vi "current monitor4.vi"() -> ()   [LabVIEW 2010]
uses:
  <vilib>/Utility/file.llb/Write To Spreadsheet File (DBL).vi
  <userlib>/Nanonis Prog Interface V5/Nanonis Prog Interface.lvlib
panel:
  out "Averaged":cluster{"f0":dbl, "df":dbl, dbl[]}(graph)
  out "Start Time":string
  in  "Number of Loops":dbl
  in  "Start":bool
  in  "Loop delay":dbl
  out "error out":errorcluster
  in  "Path":path
  out "Spectrum Analyzer":cluster{"f0":dbl, "df":dbl, "values":dbl[]}(graph)
  out "Current (A)":sgl format="%#_6p"
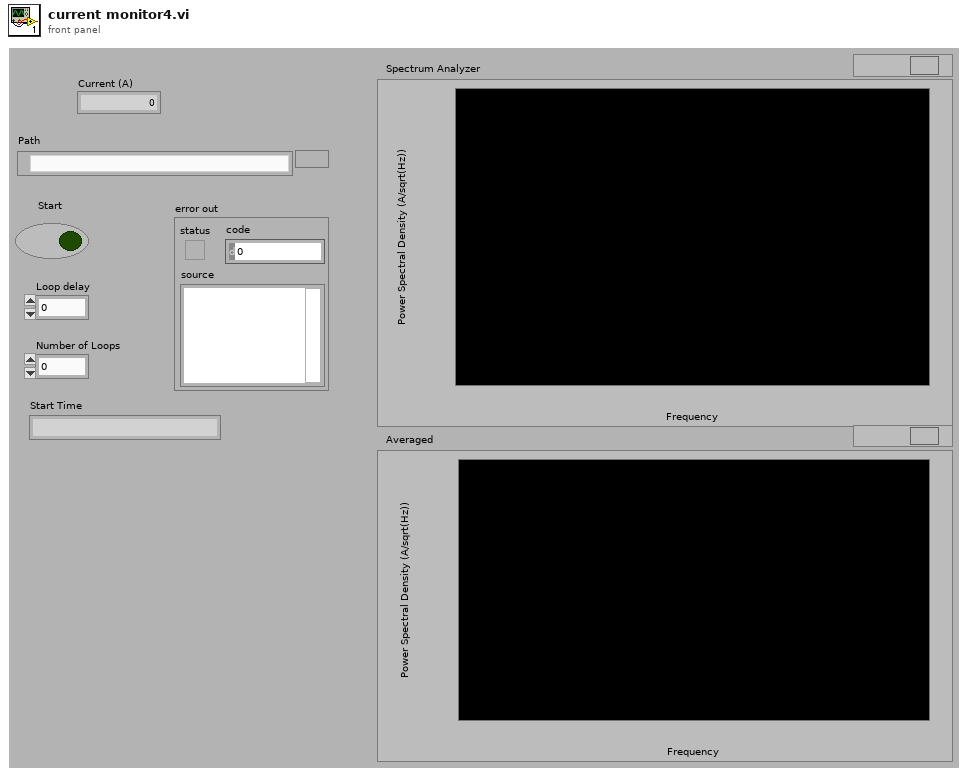
[diagram p1: front panel]
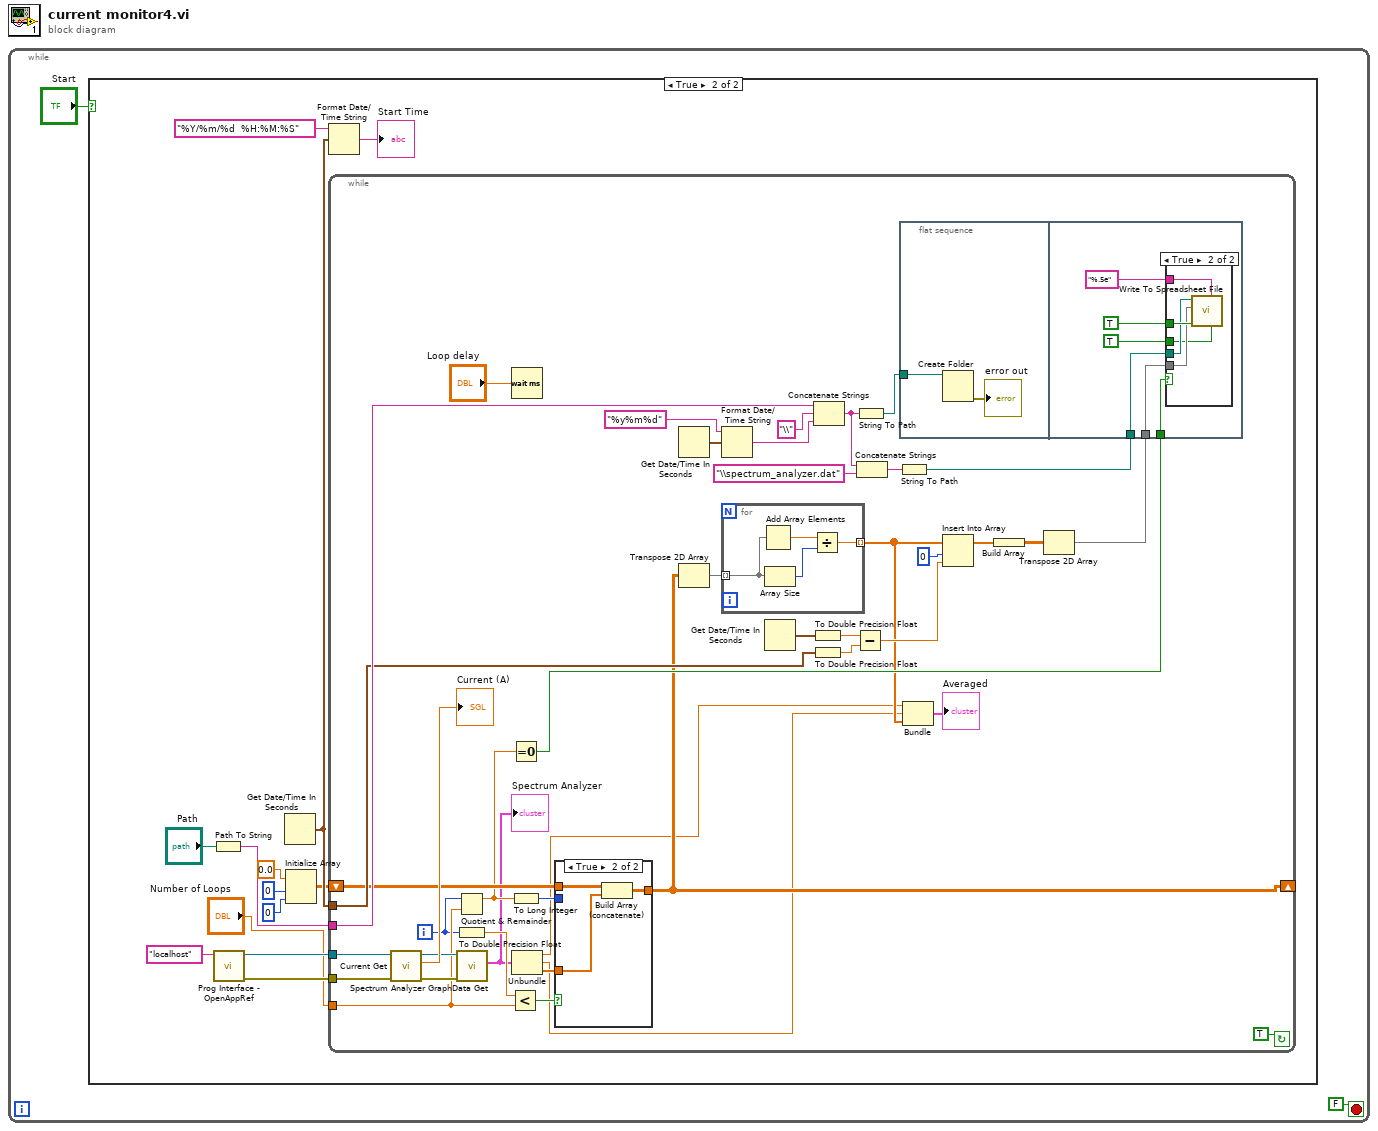
[diagram p0: block diagram]
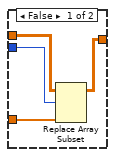
[diagram p3: hidden frame]
diagram:
  n1 = while {
    stop <- FALSE stop-if-true
    n2 = case shown="True" "Start" {
      frame False {
      }
      frame True {
        n3 = Path To String(path="Path") -> (string=w11:string)
        n4 = call <userlib>:"Prog Interface - OpenAppRef.vi"("Machine name (local machine IP)"="localhost" ("machine name (localhost)")) -> ("Error out"=w14:errorcluster, "Application reference"=w15:refnum<vi>)  [unwired: 5 in]
        n5 = Get Date/Time In Seconds() -> (seconds since 1Jan1904=w9:timestamp)
        n6 = Initialize Array(0.0, 0, 0) -> (w3:dbl[][])
        n7 = Format Date/Time String(time format string (%c)="%Y/%m/%d  %H:%M:%S", seconds (now)=w9) -> (date/time string=→"Start Time":string)  [unwired: 1 in]
        n8 = while {
          tunnel: w15 -> [w57]
          tunnel: w14 -> [w56]
          tunnel: w11 -> [w49]
          tunnel: w9 -> [w35]
          tunnel: "Number of Loops" -> [w30]
          shift-right: [w24] -> _
          shift-left: w3 -> [w27]
          i -> [w26]
          stop <- TRUE continue-if-true
          n9 = call <userlib>:"Current Get.vi"("Error in (no error)"=w56, "Application ref in"=w57) -> ("Error out"=w53:errorcluster, "Current (A)"=→"Current (A)":sgl, "Application ref out"=w54:refnum<vi>)  [unwired: 5 in]
          n10 = Quotient & Remainder(x=w26, y=w30) -> (x-y*floor(x/y)=w21:dbl)  [unwired: 1 out]
          n11 = To Double Precision Float(number=w26) -> (double precision float=w29:dbl)
          n12 = call <userlib>:"Spectrum Analyzer GraphData Get.vi"("Error in (no error)"=w53, "Application ref in"=w54) -> ("FFT data"=w20:cluster{"f0":dbl, "df":dbl, "values":dbl[]})  [unwired: 7 in, 2 out]
          "Spectrum Analyzer" <- w20
          n13 = Less?(x=w29, y=w30) -> (x < y?=w31:bool)
          n14 = Equal To 0?(x=w21) -> (x = 0?=w41:bool)
          n15 = To Long Integer(number=w21) -> (32bit integer=w22:i32)
          n16 = Wait (ms)(milliseconds to wait="Loop delay") -> ()  [unwired: 1 out]
          n17 = Unbundle(w20) -> ("f0"=w17:dbl, "df"=w16:dbl, "values"=w28:dbl[])
          n18 = case shown="True" w31 {
            tunnel: w28 -> [w63 w68]
            tunnel: [w64 w67] -> w24
            tunnel: w27 -> [w65 w66]
            tunnel: w22 -> [w62 _]
            frame False {
              n19 = Replace Array Subset(array=w65, new element=w63, index (row)=w62) -> (w64:dbl[][])  [unwired: 1 in]
            }
            frame True {
              n20 = Build Array (concatenate)(w66, w68) -> (w67:dbl[][])
            }
          }
          n21 = Get Date/Time In Seconds() -> (seconds since 1Jan1904=w50:timestamp)
          n22 = Transpose 2D Array(2D array=w24) -> (transposed array=w23:dbl[][])
          n23 = Format Date/Time String(time format string (%c)="%y%m%d", seconds (now)=w50) -> (date/time string=w47:string)  [unwired: 1 in]
          n24 = for {
            tunnel: w23 -> [w61] mode=indexing
            tunnel: [w58] -> w18 mode=indexing
            n25 = Add Array Elements(numeric array=w61) -> (sum=w60:dbl)
            n26 = Array Size(array=w61) -> (size(s)=w59:i32)
            n27 = Divide(x=w60, y=w59) -> (x/y=w58:dbl)
          }
          n28 = Get Date/Time In Seconds() -> (seconds since 1Jan1904=w38:timestamp)
          n29 = To Double Precision Float(number=w38) -> (double precision float=w37:dbl)
          n30 = To Double Precision Float(number=w35) -> (double precision float=w36:dbl)
          n31 = Concatenate Strings(w49, "\\" ("string"), w47) -> (w42:string)
          n32 = Subtract(x=w37, y=w36) -> (x-y=w39:dbl)
          n33 = String To Path(string=w42) -> (path=w48:path)
          n34 = Concatenate Strings(w42, "\\spectrum_analyzer.dat" ("string")) -> (w33:string)
          n35 = String To Path(string=w33) -> (path=w52:path)
          n36 = flat-sequence {
            tunnel: w48 -> [w70]
            tunnel: w52 -> [w73]
            tunnel: w43 -> [w74]
            tunnel: w41 -> [w72]
            frame #0 {
              n37 = Create Folder(path (use dialog)=w70) -> (error out=→"error out":errorcluster)  [unwired: 2 in, 2 out]
            }
            frame #1 {
              n38 = case shown="True" w72 {
                tunnel: TRUE ("append to file? (new file:F)") -> [_ w81]
                tunnel: "%.5e" ("format (%.3f)") -> [_ w80]
                tunnel: w74 -> [_ w79]
                tunnel: w73 -> [_ w78]
                tunnel: TRUE -> [_ w77]
                frame False {
                }
                frame True {
                  n39 = call-poly <vilib>:"Write To Spreadsheet File.vi"("transpose? (no:F)"=w77, "format (%.3f)"=w80, "append to file? (new file:F)"=w81, "2D data"=w79, "file path (dialog if empty)"=w78) -> ()  [unwired: 3 in, 1 out]
                }
              }
            }
          }
          n40 = Bundle("f0"=w17, "df"=w16, w18) -> (→"Averaged":cluster{"f0":dbl, "df":dbl, dbl[]})  [unwired: 1 in]
          n41 = Insert Into Array(array=w18, index=0, new element=w39) -> (w32:dbl[])
          n42 = Build Array(w32) -> (w44:dbl[][])
          n43 = Transpose 2D Array(2D array=w44) -> (transposed array=w43:dbl[][])
        }
      }
    }
  }
